vi "uService Probe - core.vi"(11 "Father of all uServices in":refnum<class "Father of all uServices.lvclass">) -> (2 "Value String":string, 3 "Boolean":bool)   [LabVIEW 2026, in "TALOS.lvlib" / "Father of all uServices.lvlib" / "Father of all uServices.lvclass"]
uses:
  Father of all uServices.lvclass
  Father of all uServices.lvclass/Father of all uServices.ctl
  Classes/Config/Config.lvclass
panel:
  out "Config":map{string, map{string, string}}(c390)
  out "Safe Mode":bool
  out "uService Class Name":string
  out "uService ID":string
  in  "uService ID to check":string caption="uService ID for comparison"
  # "="
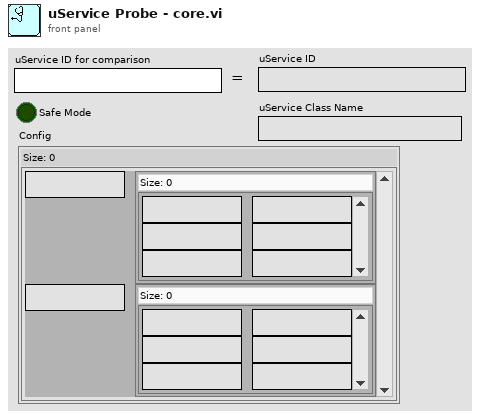
[diagram p1: front panel]
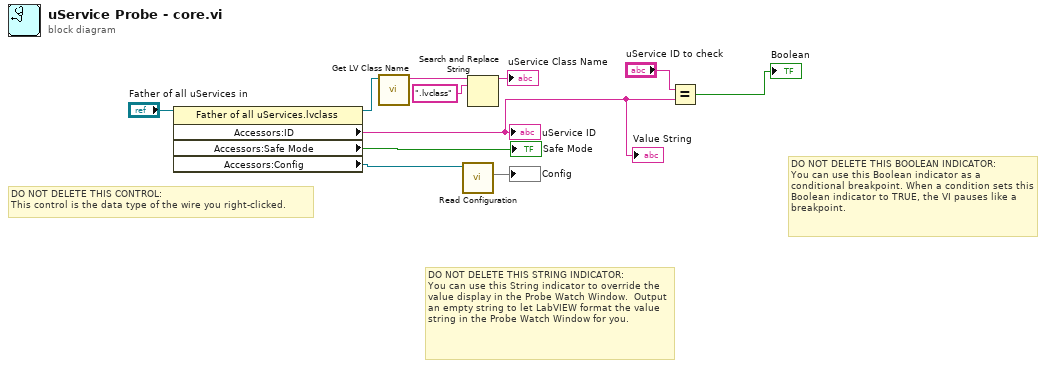
[diagram p0: block diagram]
diagram:
  # "DO NOT DELETE THIS STRING INDICATOR: \nYou can use this String indicator to override the value display in the Probe Watch Window.  Output an empty string to let LabVIEW format the value string in the Probe Watch Window for you."
  # "DO NOT DELETE THIS BOOLEAN INDICATOR: \nYou can use this Boolean indicator as a conditional breakpoint. When a condition sets this Boolean indicator to TRUE, the VI pauses like a breakpoint."
  # "DO NOT DELETE THIS CONTROL: \nThis control is the data type of the wire you right-clicked."
  n1 = property class="Father of all uServices.lvclass"(reference="Father of all uServices in") -> (reference out=w2:refnum<class "Father of all uServices.lvclass">, "Accessors:ID"=w1:string, "Accessors:Safe Mode"=→"Safe Mode":bool, "Accessors:Config"=w4:refnum<class "Config.lvclass">)  [unwired: 1 in, 1 out]
  "Value String" <- w1
  "uService ID" <- w1
  n2 = call <vilib>:"Get LV Class Name.vi"("object"=w2) -> ("class name"=w10:string)  [unwired: 9 in, 1 out]
  n3 = call "Read Configuration.vi"("Config in"=w4) -> ("Configuration"=→"Config":map{string, map{string, string}})  [unwired: 8 in, 2 out]
  n4 = Search and Replace String(input string=w10, search string=".lvclass") -> (result string=→"uService Class Name":string)  [unwired: 6 in, 3 out]
  n5 = Equal?(x="uService ID to check", y=w1) -> (x = y?=→"Boolean":bool)
